vi "CMN_toDBS.vi"(6 "ms timeout (-1)":i32=-1, 8 "error in (no error)":errorcluster, 9 "response Q":string, 11 "command":string) -> (0 "error out":errorcluster, 1 "timeout":bool, 2 "response":string)   [LabVIEW 2016]
panel:
  in  "cmdstruct":cluster{"command":string, "respond to":string}
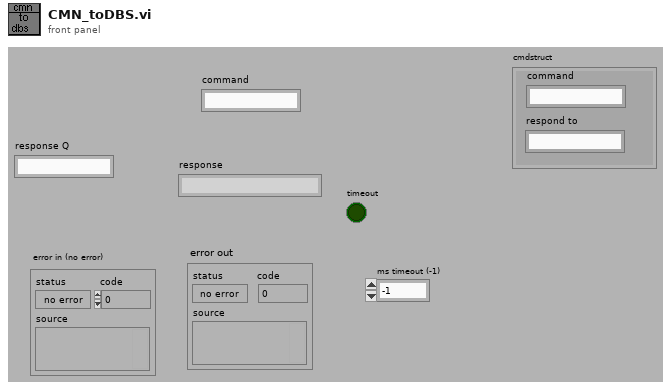
[diagram p1: front panel]
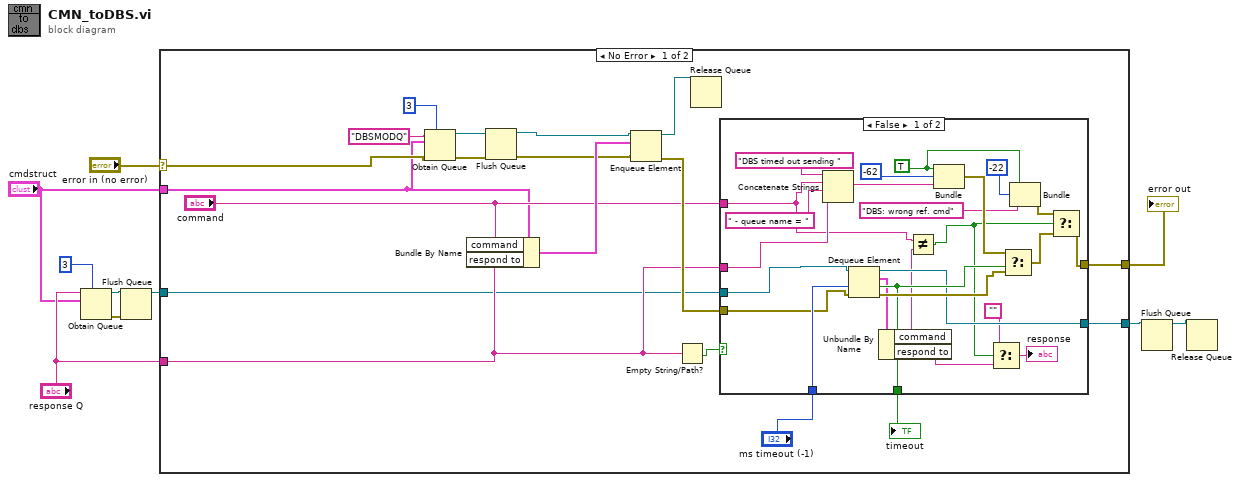
[diagram p0: block diagram]
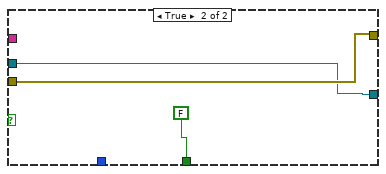
[diagram p2: hidden frame]
diagram:
  n1 = Obtain Queue(max queue size (-1, unlimited)=3, name (unnamed)="response Q", element data type="cmdstruct") -> (queue out=w6:refnum<queue>, error out=w7:errorcluster)  [unwired: 2 in, 1 out]
  n2 = Flush Queue(queue=w6, error in (no error)=w7) -> (queue out=w5:refnum<queue>)  [unwired: 2 out]
  n3 = case shown="No Error" "error in (no error)" {
    selector: "error in (no error)" -> [w24 w59]
    tunnel: [w26 w59] -> w9
    tunnel: "response Q" -> [w16 _]
    tunnel: w5 -> [w15 w58]
    tunnel: [w14 w58] -> w3
    tunnel: "cmdstruct" -> [w12 _]
    frame No Error {
      n4 = Obtain Queue(max queue size (-1, unlimited)=3, name (unnamed)="DBSMODQ", element data type=w12, error in (no error)=w24) -> (queue out=w19:refnum<queue>, error out=w20:errorcluster)  [unwired: 1 in, 1 out]
      n5 = Bundle By Name(cluster=w12, "command"="command", "respond to"=w16) -> (w25:cluster{"command":string, "respond to":string})
      n6 = Flush Queue(queue=w19, error in (no error)=w20) -> (queue out=w18:refnum<queue>, error out=w17:errorcluster)  [unwired: 1 out]
      n7 = Enqueue Element(queue=w18, element=w25, error in (no error)=w17) -> (queue out=w13:refnum<queue>, error out=w23:errorcluster)  [unwired: 2 out]
      n8 = Empty String/Path?(string/path=w16) -> (empty?=w28:bool)
      n9 = Release Queue(queue=w13) -> ()  [unwired: 1 in, 4 out]
      n10 = case shown="False" w28 {
        tunnel: w16 -> [w49 _]
        tunnel: "ms timeout (-1)" -> [w48 _]
        tunnel: w23 -> [w44 w57]
        tunnel: [w35 w57] -> w26
        tunnel: "command" -> [w40 _]
        tunnel: [w46 FALSE ("timed out?")] -> w21
        tunnel: w15 -> [w45 w55]
        tunnel: [w43 w55] -> w14
        frame False {
          w38 = TRUE
          n11 = Concatenate Strings("DBS timed out sending " ("source"), w40, " - queue name = ", w49) -> (w52:string)
          n12 = Dequeue Element(queue=w45, timeout in ms (-1)=w48, error in (no error)=w44) -> (queue out=w43:refnum<queue>, element=w42:cluster{"command":string, "respond to":string}, timed out?=w46:bool, error out=w47:errorcluster)
          n13 = Unbundle By Name(w42) -> ("command"=w41:string, "respond to"=w32:string)
          n14 = Not Equal?(x=w40, y=w41) -> (x != y?=w33:bool)
          n15 = Bundle(w38, -62, w52) -> (w53:errorcluster)  [unwired: 1 out]
          n16 = Select(t="", s=w33, f=w32) -> (s? t:f=→"response":string)
          n17 = Select(t=w53, s=w46, f=w47) -> (s? t:f=w34:errorcluster)
          n18 = Bundle(w38, -22, "source"="DBS: wrong ref. cmd") -> (w39:cluster{bool, i32, "source":string})  [unwired: 1 out]
          n19 = Select(t=w39, s=w33, f=w34) -> (s? t:f=w35:errorcluster)
        }
        frame True {
        }
      }
      "timeout" <- w21
    }
    frame Error {
    }
  }
  "error out" <- w9
  n20 = Flush Queue(queue=w3) -> (queue out=w4:refnum<queue>)  [unwired: 1 in, 2 out]
  n21 = Release Queue(queue=w4) -> ()  [unwired: 1 in, 4 out]
